vi "Save CalCfg File Data.vi"(6 "Matric Section":string[](array[string]), 8 "error in":errorcluster, 10 "File Path":path, 11 "Config Data":T1(array[cluster])) -> (0 "error out":errorcluster)   [LabVIEW 2020, in "GUCalibration2.lvlib"]
uses:
  GUCalibration2.lvlib
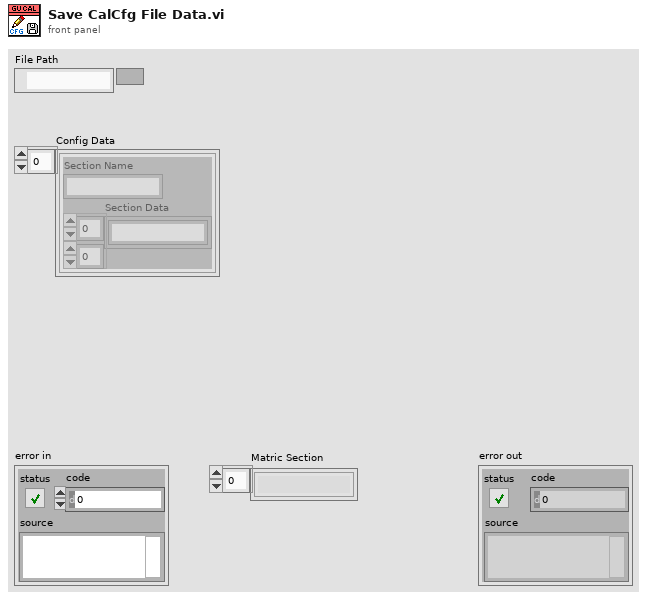
[diagram p1: front panel]
types:
  T1 = cluster{"Section Name":string, "Section Data":string[][]}[]
  T2 = enum16{"open", "replace", "create", "open or create", "replace or create", "replace or create with confirmation"}
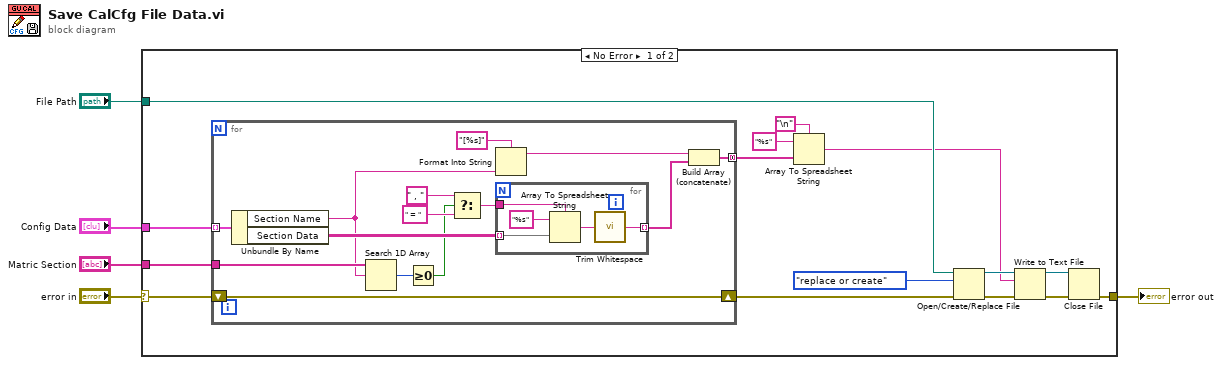
[diagram p0: block diagram]
diagram:
  n1 = case shown="No Error" "error in" {
    selector: "error in" -> [w6 w40]
    tunnel: "Config Data" -> [w20 _]
    tunnel: "Matric Section" -> [w19 _]
    tunnel: [w9 w40] -> w3
    tunnel: "File Path" -> [w8 _]
    frame No Error {
      n2 = for {
        tunnel: w20 -> [w34] mode=indexing
        tunnel: [w27] -> w16 mode=concatenating
        shift-right: [w21] -> w10
        shift-left: w6 -> [w21]
        tunnel: w19 -> [w25]
        n3 = Unbundle By Name(w34) -> ("Section Name"=w24:string, "Section Data"=w32:string[][])
        n4 = Search 1D Array(1D array=w25, element=w24) -> (index of element=w23:i32)  [unwired: 1 in]
        n5 = Greater Or Equal To 0?(x=w23) -> (x >= 0?=w22:bool)
        n6 = Select(t=" , " ("format string"), s=w22, f=" = " ("format string")) -> (s? t:f=w29:string)
        n7 = Format Into String(format string="[%s]", w24) -> (resulting string=w26:string)  [unwired: 2 in, 1 out]
        n8 = for {
          tunnel: w32 -> [w39] mode=indexing
          tunnel: w29 -> [w37]
          tunnel: [w36] -> w28 mode=indexing
          n9 = Array To Spreadsheet String(delimiter (Tab)=w37, array=w39, 3:"%s" ("format string")) -> (spreadsheet string=w35:string)
          n10 = call <vilib>:"Trim Whitespace.vi"("string"=w35) -> ("trimmed string"=w36:string)  [unwired: 1 in]
        }
        n11 = Build Array (concatenate)(w26, w28) -> (w27:string[])
      }
      n12 = Array To Spreadsheet String(delimiter (Tab)="\n", array=w16, 3:"%s" ("format string")) -> (spreadsheet string=w7:string)
      n13 = Open/Create/Replace File(file path (use dialog)=w8, error in=w10, operation (0:open)=T2."replace or create") -> (refnum out=w13:refnum<file>, error out=w14:errorcluster)  [unwired: 3 in, 1 out]
      n14 = Write to Text File(file (use dialog)=w13, text=w7, error in=w14) -> (refnum out=w12:refnum<file>, error out=w11:errorcluster)  [unwired: 1 in, 1 out]
      n15 = Close File(refnum=w12, error in=w11) -> (error out=w9:errorcluster)  [unwired: 1 out]
    }
    frame Error {
    }
  }
  "error out" <- w3
